vi "TrapControllers.vi"() -> ()   [LabVIEW 2016]
doc: "I. Description:\nThis example demonstrates how to continuously output a waveform using an internal sample clock. The automatic regeneration of data has been disabled, so new data has to be provided throughout the duration of the continuous Analog Output operation. This allows the generation of any arbitrary frequency as this VI computes new data for each iteration of the loop, maintaining phase continuity of the signal. The regeneration of data has also been adjusted so that the newest data is output as quickly as possible; thus reducing the lag between the changing of the data and the output of that data.\n\nII. Instructions for Running:\n1. Select the Physical Channel to correspond to where your signal is output on the DAQ device.\n2. Enter the Minimum and Maximum Voltage range.\n3. Specify the desired Sample Clock Rate of the output Waveform. Higher sample clock rates will produce a smoother waveform.\n4. Manually specify the Analog Output buffer size, in number of samples. A larger buffer would help non-regenerative operations avoid errors due to occasional high CPU load. \nNote: \nThe Analog Output buffer has to be at least as big as the amount of data being written to the board per iteration. The recommended buffer size would be at least twice the amount of data being written to the board per iteration.\n5. Enter the Waveform Information. See the documentation of the Basic Function Generator SubVI for information on each parameter.\n\nIII. Block Diagram Steps:\n1. Create an Analog Output Voltage channel.\n2. Configure the task to prohibit the automatic regeneration of data.\n2a. Set the transfer condition to Less than Full. Allows for more rapid updates of Output Buffer.\n3. Call the DAQmx (Sample Clock) VI to set the sample clock rate. Additionally, set the sample mode to Continuous.\n4. Read the actual sample clock rate (eventually coerced depending on the hardware used). \n5. Compute the desired waveform, using the buffer size and the actual update rate. This VI keeps track of the phase of the waveform to ensure that the generated signal is continuous.\n6. Write the waveform to the output buffer. \n7a. Call the Start VI. This is only needed when the loop is executed for the first time.\n7b. Do nothing.\n8. Loop continuously until user presses the Stop button. Every iteration computes and writes a new waveform to the buffer.\n9. Call the Clear Task VI to clear the Task.\n10. Use the popup dialog box to display an error or warning if any.\n\nIV. I/O Connections Overview:\nMake sure your signal output terminal matches the Physical Channel I/O Control. For further connection information, refer to your hardware reference manual."
uses:
  <vilib>/event_ctls.llb/eventvkey.ctl
  <vilib>/DAQmx/write.llb/DAQmx Write (Digital 1D Bool NChan 1Samp 1Line).vi
  <vilib>/DAQmx/write.llb/DAQmx Write (Analog DBL 1Chan 1Samp).vi
  <vilib>/DAQmx/write.llb/DAQmx Write (Analog 1D DBL NChan 1Samp).vi
  <vilib>/DAQmx/create/channels.llb/DAQmx Create Channel (DO-Digital Output).vi
  <vilib>/DAQmx/miscellaneous.llb/DAQmx Fill In Error Info.vi
  <vilib>/DAQmx/create/channels.llb/DAQmx Create Channel (AO-Voltage-Basic).vi
  PZT_PI/PZT_oscillation.vi
panel:
  in  "VISA resource name":refnum<visa-resource-name>
  out "Off":string
  out "Error 2":string
  out "On":string
  out "Move":string
  in  "Move":bool
  in  "Query?":bool
  in  "Step":i32 min=0 max=10 step=1
  out "Status":string
  out "Position":string
  out "Error":string
  in  "StageZ_Start":bool
  in  "StageY_Start":bool
  out "StageY_Connection":bool
  in  "StageY_Home":bool
  out "StageY_Position":dbl caption="Pos (um)" format="%.1f"
  in  "StageY_Step2":dbl=1.0 caption="Step2" min=0.0 max=1000.0 step=0.1 format="%.1f"
  in  "StageY_Step1":dbl=10.0 caption="Step1" min=0.0 max=1000.0 step=0.1 format="%.1f"
  out "StageY_Step":dbl=10.0 caption="Step (um)" min=0.0 max=1000.0 step=0.1 format="%.1f"
  out "VKey":T1
  out "Char":i16
  out "ScanCode":i16
  out "StageX_Step":dbl=10.0 caption="Step (um)" min=0.0 max=1000.0 step=0.1 format="%.1f"
  in  "StageX_Step2":dbl=1.0 caption="Step2" min=0.0 max=1000.0 step=0.1 format="%.1f"
  in  "Stage_Step_Select":bool=TRUE
  out "Numeric":i32
  out "StageX_Connection":bool
  in  "StageZ_Stop":bool
  in  "StageY_Stop":bool
  in  "StageX_Stop":bool
  in  "StageZ-":bool
  in  "StageZ+":bool
  in  "StageY-":bool
  in  "StageY+":bool
  in  "StageX+":bool
  in  "StageX-":bool
  out "StageY_Limit 2":bool caption="Limit"
  out "StageY_Limit":bool caption="Limit"
  out "StageX_Limit":bool caption="Limit"
  out "PZT_Error 6":bool
  out "PZT_Error 5":bool
  out "PZT_Error 4":bool
  out "PZT_Error 3":bool
  out "PZT_Error 2":bool
  out "PZT_Error":bool
  in  "StageX_Step1":dbl=10.0 caption="Step1" min=0.0 max=1000.0 step=0.1 format="%.1f"
  in  "StageX_Home":bool
  out "?":i32
  out "?":i32
  out "PZT_Z 2":dbl caption="Z"
  out "StageX_Position":dbl caption="Pos (um)" format="%.1f"
  in  "StageX_Start":bool
  in  "PZT_Step":dbl=10.0 caption="Step (nm)" min=0.0 max=1000.0 step=1.0
  in  "Flu_Red_Power":dbl=1.0 caption="(%)" min=0.0 max=100.0 step=1.0
  in  "Flu_Green_Power":dbl=1.0 caption="(%)" min=0.0 max=100.0 step=1.0
  in  "Flu_Blue_Power":dbl=1.0 caption="(%)" min=0.0 max=100.0 step=1.0
  in  "Flu_Red":bool caption="640"
  in  "Flu_Green":bool caption="561"
  in  "Flu_Blue":bool caption="488"
  in  "stop 6":bool
  out "Numeric 9":i32
  out "OK Button 10":bool
  in  "OK Button 6":bool
  in  "Trap_control 2":dbl=1.0 caption="Power (%)" min=1.0 max=10.0 step=0.1 format="%.1f"
  in  "Detection_Feedback":bool caption="Feedback"
  in  "Detection_ON":bool caption="ON/OFF (d)"
  in  "stop 4":bool
  out "Numeric 7":i32
  in  "OK Button 4":bool
  out "OK Button 8":bool
  in  "stop 5":bool
  out "Numeric 8":i32
  in  "OK Button 5":bool
  out "OK Button 9":bool
  in  "Trap_Feedback":bool caption="Feedback"
  in  "Trap_ON":bool caption="ON/OFF (t)"
  in  "Trap_control":dbl=1.0 caption="Power (%)" min=1.0 max=100.0 step=1.0
  in  "Trap_STOP1":bool
  out "Numeric 5":i32
  in  "Trap_START1":bool
  out "Trap_START2":bool
  in  "PZT_oscillation":bool caption="Start\n(Ctrl)"
  out "PZT_os_num":i32
  out "PZT_manual":bool
  in  "PZT_Amplitude":dbl=10.0 caption="Amp (nm)" min=0.0 max=100.0 step=1.0
  in  "PZT_Frequency":dbl=1.0 caption="Freq (Hz)" min=0.0 max=100.0 step=1.0
  in  "PZT_Waveform":T2(ring) caption="Waveform"
  in  "PZT_Axis":enum16{"X-axis", "Y-axis", "Z-axis"}(ring) caption="Axis"
  in  "PZTZ_move":dbl caption="Z" min=-3000.0 max=3000.0 step=1.0
  in  "PZTY_move":dbl caption="Y" min=-5000.0 max=5000.0 step=1.0
  in  "PZTX_move":dbl caption="X" min=-5000.0 max=5000.0 step=1.0
  out "PZTZ_Vin":dbl format="%.5f"
  out "PZTY_Vin":dbl format="%.5f"
  out "PZTX_Vin":dbl format="%.5f"
  out "PZT_Z":dbl caption="Z"
  out "PZT_Y":dbl caption="Y"
  out "PZT_X":dbl caption="X"
  in  "PZT_Move":bool
  out "PZT_Caution":bool caption="Limit"
  in  "PZT_Time":dbl=100.0 caption="Vel (%)" min=0.0 max=100.0 step=1.0
  in  "PZT_Center":bool
  in  "PZT_Z-":bool
  in  "PZT_Z+":bool
  in  "PZT_Y-":bool
  in  "PZT_Y+":bool
  in  "PZT_X+":bool
  in  "PZT_X-":bool
  out "PZT_ON":bool
  in  "PZT_START":bool
  out "PZT_man_num":i32
  in  "PZT_STOP":bool
  in  "STOP":bool
  # "Stop sub-programs first >> STOP PROGRAM"
  # "Servo should be ON.\nProgram START -> PZT power ON\nRange: X/Y = +/- 5 um, Z = +/- 3 um"
  # "Stage"
  # "PZT"
  # "Range: X/Y = +/- 2.5 mm"
  # "Move to"
  # "Pos (nm)"
  # "Vin (V)"
  # "Manual"
  # "Oscillation"
  # "Feedback"
  # "1 = 10 nm"
  # "Trap Laser"
  # "Detection Laser"
  # "Fluorescent Laser"
  # "Template"
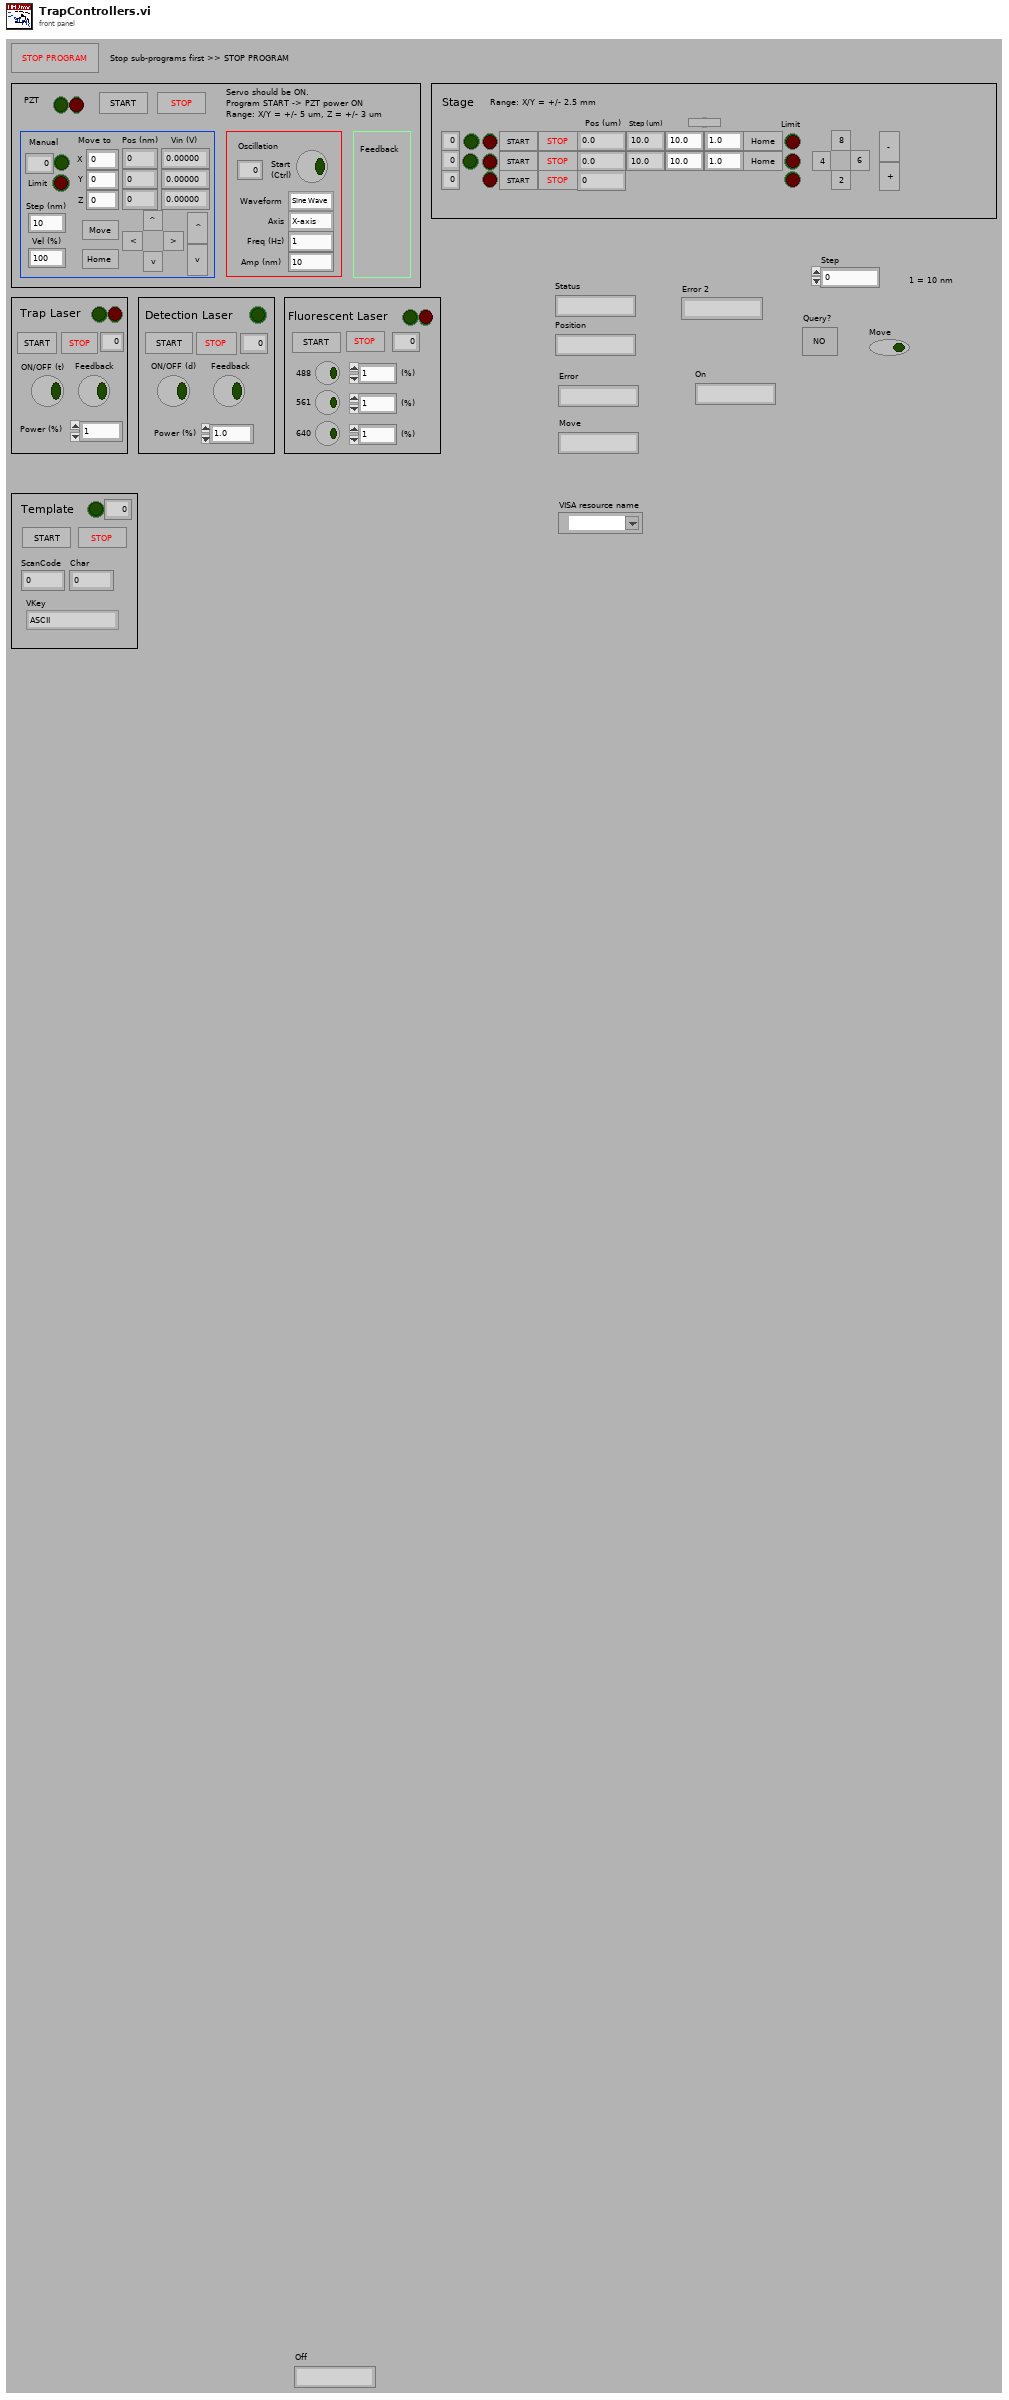
[diagram p1: front panel]
types:
  T1 = typedef "eventvkey.ctl" = enum16{"ASCII", "Enter", "Return", "Shift", "Ctrl", "Alt", "Cmd", "Opt", "Caps", "NumLock", "Clear", "Break", "Up", "Down", "Left", "Right", "Insert", "Delete", "Home", "End", "PageUp", "PageDown", "Escape", "Help", "Pause", "ScrollLock", "F1", "F2", "F3", "F4", "F5", "F6", "F7", "F8", "F9", "F10", "F11", "F12", "F13", "F14", "F15", "F16", "F17", "F18", "F19", "F20", "F21", "F22", "F23", "F24", "Play", "VolumeUp", "VolumeDown", "Mute", "Two Byte Char"}
  T2 = enum16{"Sine Wave", "Triangle Wave", "Square Wave", "Sawtooth Wave"}
  T3 = cluster{"VISA resource name":refnum<visa-resource-name>, "Device name":string, "Controller address":i32, "error":errorcluster}
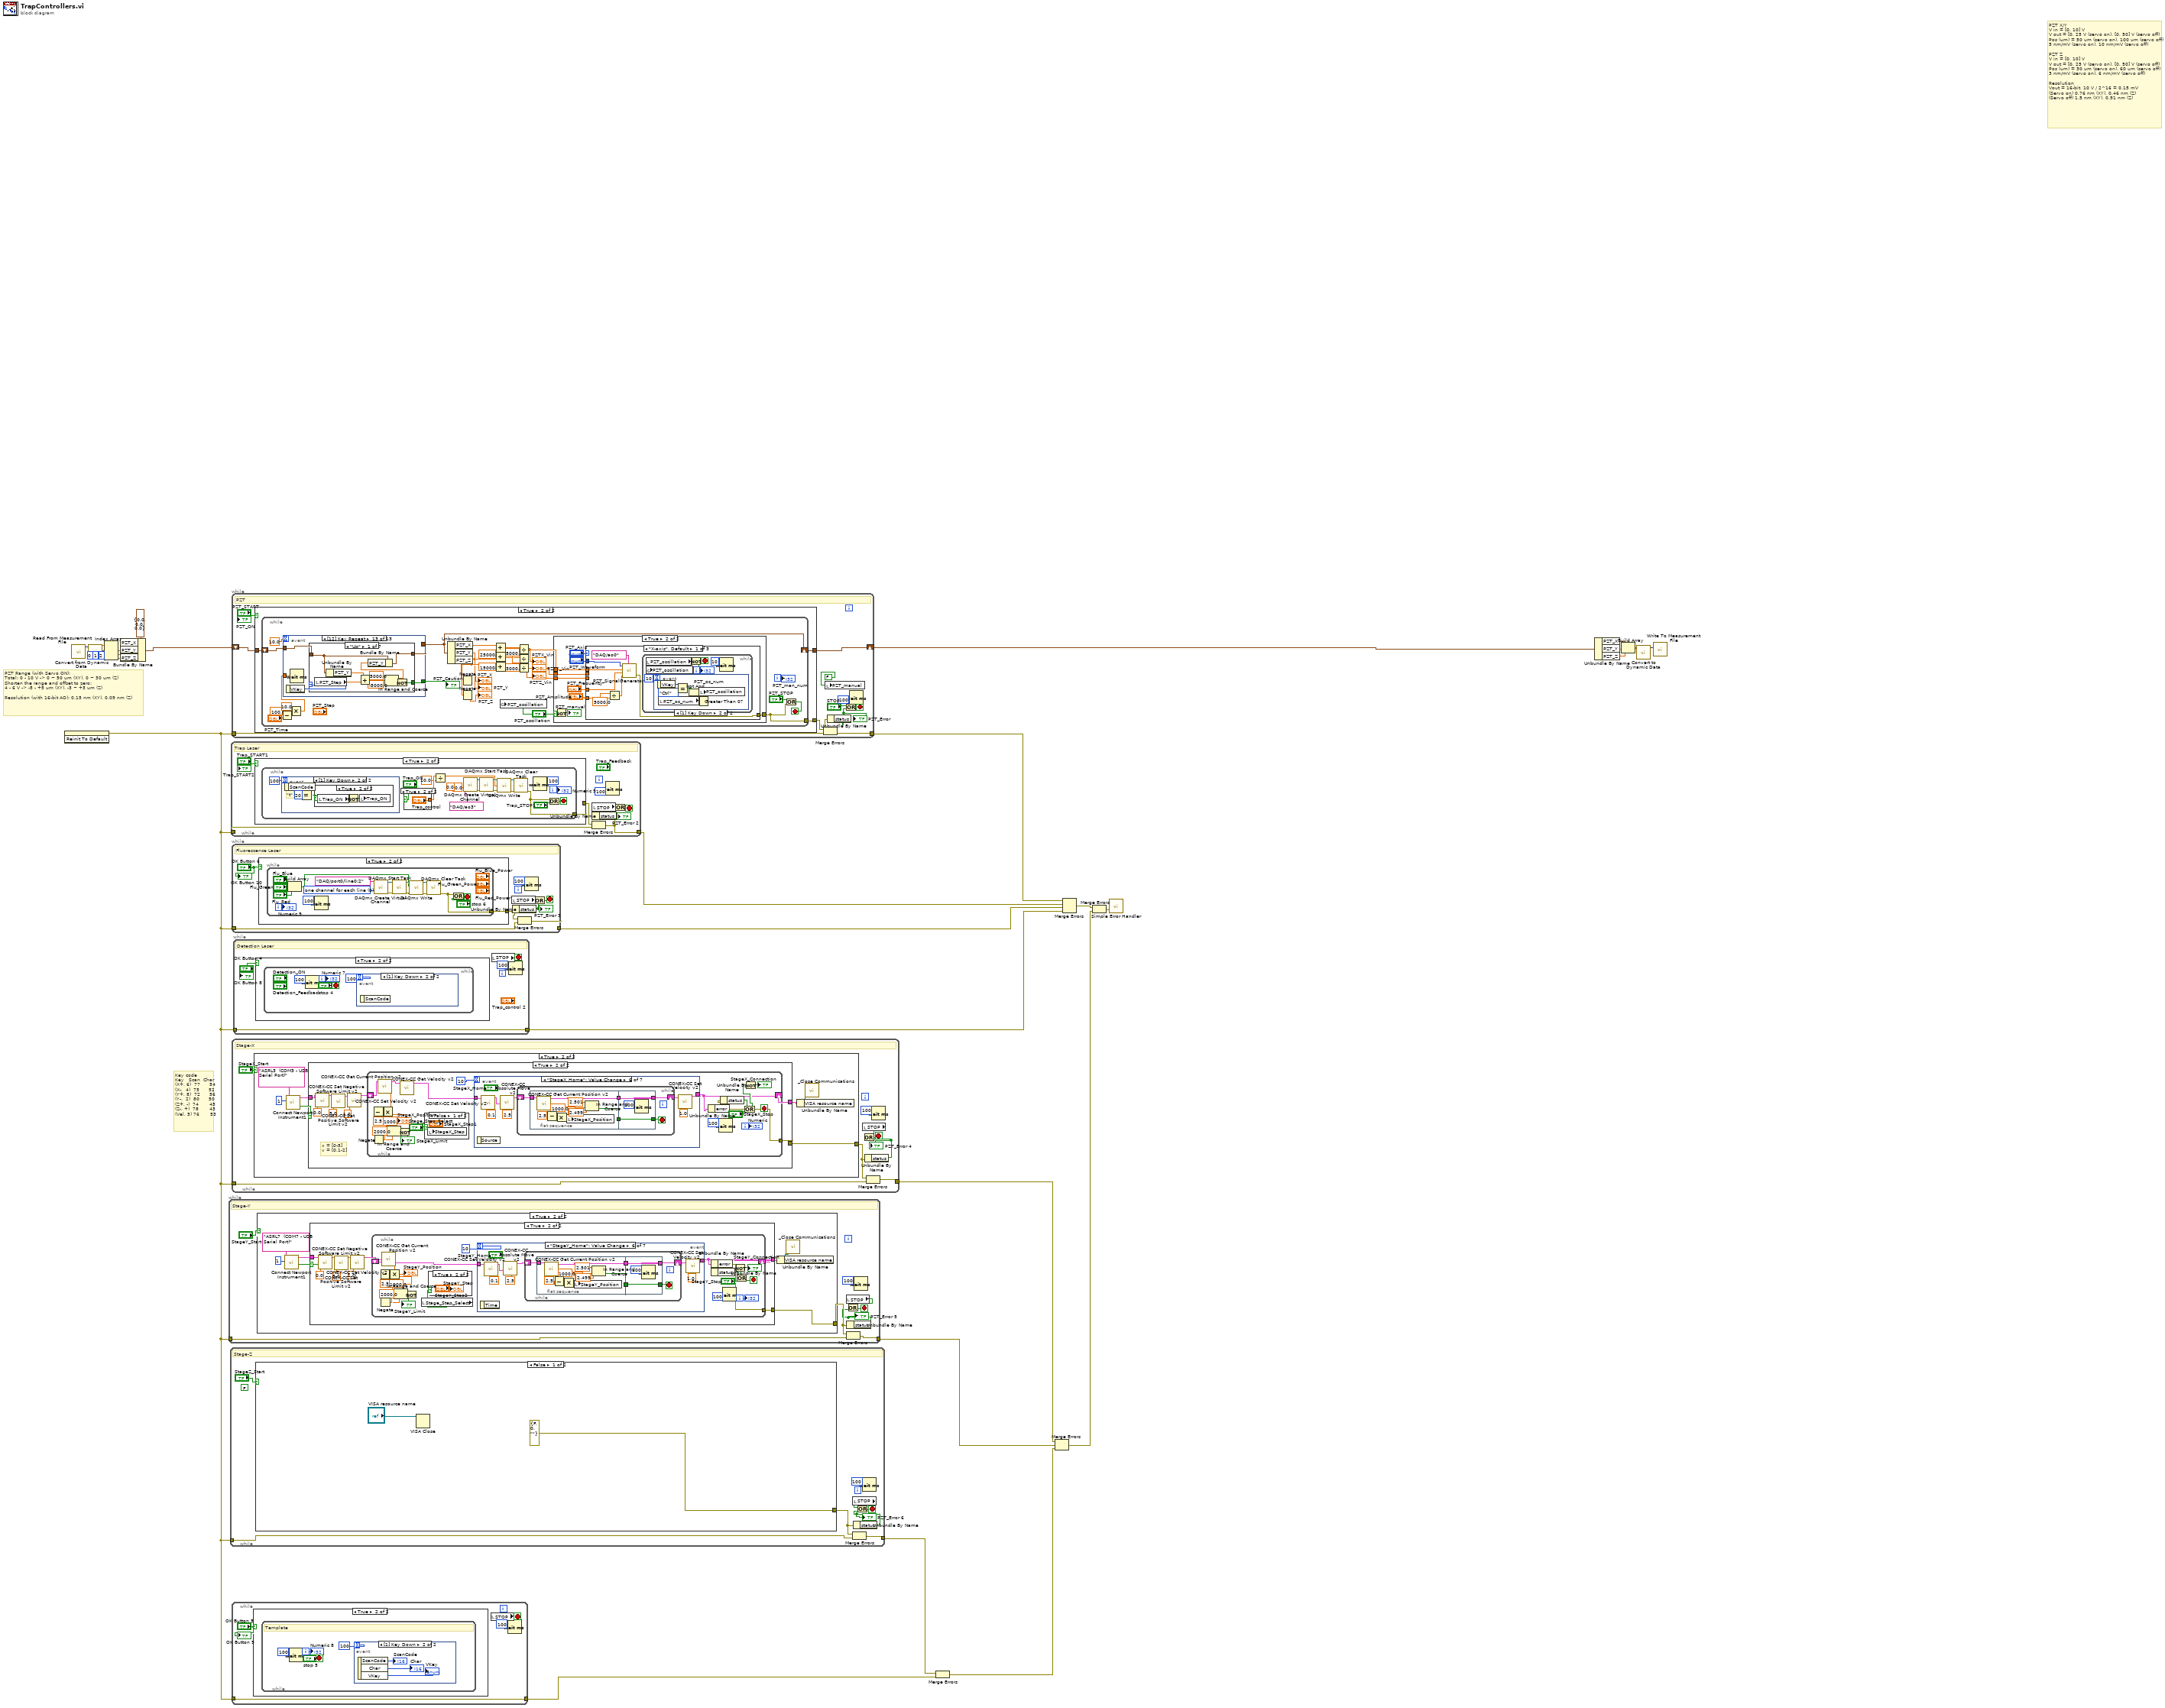
[diagram p0: block diagram]
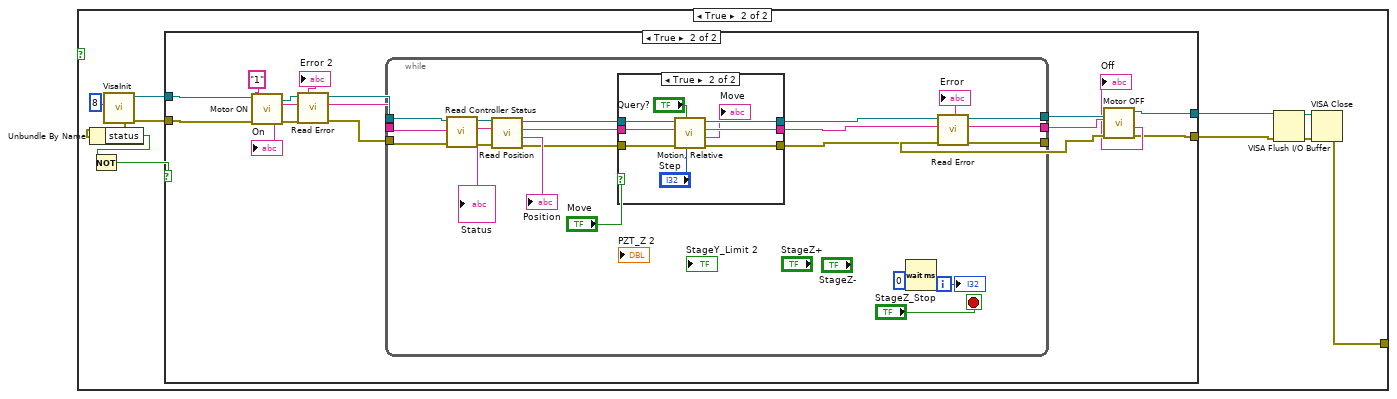
[diagram p2: hidden frame]
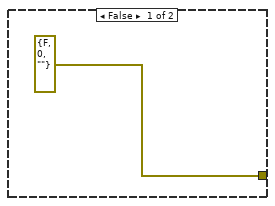
[diagram p5: hidden frame]
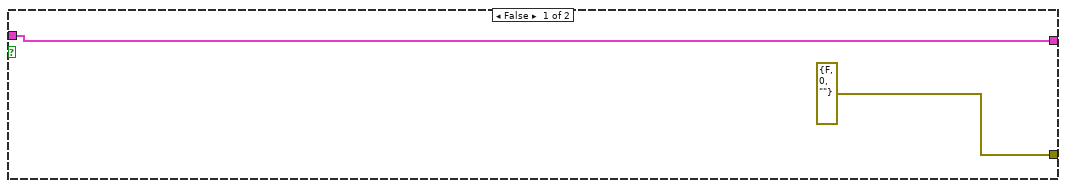
[diagram p6: hidden frame]
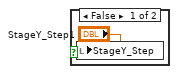
[diagram p7: hidden frame]
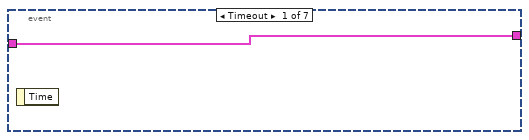
[diagram p8: hidden frame]
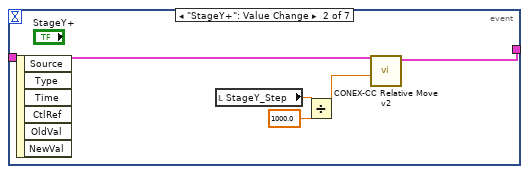
[diagram p9: hidden frame]
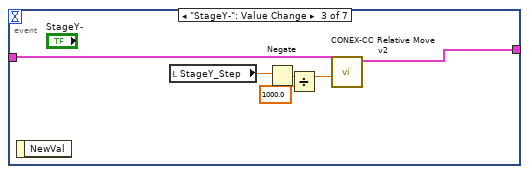
[diagram p10: hidden frame]
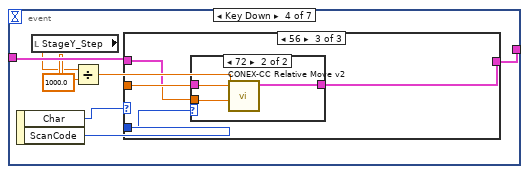
[diagram p11: hidden frame]
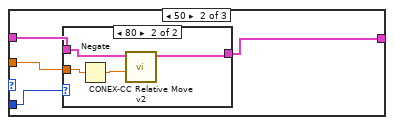
[diagram p13: hidden frame]
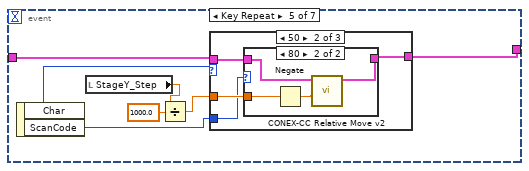
[diagram p16: hidden frame]
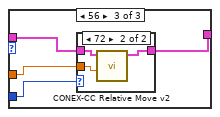
[diagram p19: hidden frame]
diagram:
  # "Key code\nKey   Scan  Char\n(X+, 6)  77      54\n(X-,  4)  75      52\n(Y+, 8)  72      56\n(Y-,  2)  80      50\n(Z+, -)  74       45\n(Z-, +)  78       43\n(Vel, 5) 76       53"
  # "PZT Range (with Servo ON):\nTotal: 0 - 10 V -> 0 ~ 50 um (XY), 0 ~ 30 um (Z)\nShorten the range and offset to zero: \n4 - 6 V -> -5 - +5 um (XY), -3 ~ +3 um (Z)\n\nResolution (with 16-bit AO): 0.15 nm (XY), 0.09 nm (Z)"
  # "PZT X/Y\nV in = [0, 10] V\nV out = [0, 25 V (servo on), [0, 50] V (servo off)\nPos (um) = 50 um (servo on), 100 um (servo off)\n5 nm/mV (servo on), 10 nm/mV (servo off)\n\nPZT Z\nV in = [0, 10] V\nV out = [0, 25 V (servo on), [0, 50] V (servo off)\nPos (um) = 30 um (servo on), 60 um (servo off)\n3 nm/mV (servo on), 6 nm/mV (servo off)\n\nResolution\nVout = 16-bit, 10 V / 2^16 = 0.15 mV\n(Servo on) 0.76 nm (XY), 0.46 nm (Z)\n(Servo off) 1.5 nm (XY), 0.91 nm (Z)"
  n1 = invoke on="STOP" class="Bool (strict)" method="Reinit To Default"() -> (error out=w2:errorcluster)  [unwired: 3 in, 2 out]
  n2 = call "Read From Measurement File"() -> ("Signals"=w26:dynamicdata)  [unwired: 6 in, 5 out]
  n3 = call "Convert from Dynamic Data"("Dynamic Data Type"=w26) -> ("Array"=w25:dbl[])  [unwired: 3 in]
  n4 = Index Array(array=w25, index #1=0 ("index"), index #2=1 ("index"), index #3=2 ("index")) -> (element #1=w21:dbl, element #2=w20:dbl, element #3=w19:dbl)
  n5 = Bundle By Name(cluster=cluster{"PZT_X":dbl, "PZT_Y":dbl, "PZT_Z":dbl} {"PZT_X"=0.0, "PZT_Y"=0.0, "PZT_Z"=0.0} ("output cluster"), "PZT_X"=w21, "PZT_Y"=w20, "PZT_Z"=w19) -> (w12:cluster{"PZT_X":dbl, "PZT_Y":dbl, "PZT_Z":dbl})
  n6 = while {
    tunnel: w2 -> [w36]
    tunnel: [w35] -> w9
    stop <- w32 stop-if-true
    # "Stage-Y"
    n7 = case shown="True" "StageY_Start" {
      tunnel: [errorcluster {"status"=FALSE, "code"=0, "source"=""} ("error out") w40] -> w34
      frame False {
      }
      frame True {
        n8 = call <userlib>:"Connect Newport Instrument1.vi"("Controller address"=1, "Selected device"="ASRL7  (COM7 - USB Serial Port)" ("String")) -> ("Connected"=w44:bool, "Device Connection Cluster"=w43:T3)  [unwired: 5 in, 3 out]
        n9 = case shown="True" w44 {
          tunnel: w43 -> [w47 w51]
          tunnel: [w47 w50] -> w41
          tunnel: [errorcluster {"status"=FALSE, "code"=0, "source"=""} ("error") w49] -> w40
          frame False {
          }
          frame True {
            n10 = call <userlib>:"CONEX-CC Set Negative Software Limit v2.vi"("Negative limit (left)"=0.0, "Connection Cluster in"=w51) -> ("Connection Cluster out"=w56:T3)  [unwired: 9 in]
            n11 = call <userlib>:"CONEX-CC Set Positive Software Limit v2.vi"("Positive limit (right)"=5.0, "Connection Cluster in"=w56) -> ("Connection Cluster out"=w55:T3)  [unwired: 9 in]
            n12 = call <userlib>:"CONEX-CC Set Velocity v2.vi"("Velocity"=1.0, "Connection Cluster in"=w55) -> ("Connection Cluster out"=w48:T3)  [unwired: 9 in]
            n13 = while "Event Handle Loop" {
              shift-right: [w64] -> w50
              shift-left: w48 -> [w68]
              tunnel: [w59] -> w49
              i -> [w76]
              stop <- w61 stop-if-true
              w74 = 2000.0 ("upper limit")
              # "Stage-Y"
              n14 = Negate(x=w74) -> (-x=w75:dbl)
              n15 = call <userlib>:"CONEX-CC Get Current Position v2.vi"("Connection Cluster in"=w68) -> ("Current position"=w69:dbl, "Connection Cluster out"=w66:T3)  [unwired: 8 in, 1 out]
              n16 = Subtract(x=w69, y=2.5) -> (x-y=w71:dbl)
              n17 = Multiply(x=w71, y=1000.0) -> (x*y=w58:dbl)
              "StageY_Position" <- w58
              n18 = In Range and Coerce(upper limit=w74, x=w58, lower limit=w75) -> (In Range?=w73:bool)  [unwired: 1 out]
              n19 = Not(x=w73) -> (.not. x?=→"StageY_Limit":bool)
              n20 = local read "Stage_Step_Select"() -> (w57:bool)
              n21 = case shown="True" w57 {
                frame False {
                  n22 = local write "StageY_Step"("StageY_Step1") -> ()
                }
                frame True {
                  "StageY_Step" <- "StageY_Step2"
                }
              }
              n23 = event shown="[5] \"StageY_Home\": Value Change" {
                selector: _ -> [_ _ _ _ _ _ _]
                dyn-events: _ -> [_ _ _ _ _ _ _]
                timeout: 10 -> [_ _ _ _ _ _ _]
                tunnel: w66 -> [w80 w81 w91 w98 w123 w149 w171]
                tunnel: [w80 w85 w88 w97 w122 w142 w171] -> w64
                event Timeout {
                  n24 = event-data() -> ()  [unwired: 1 in, 1 out]
                }
                event "StageY+": Value Change {
                  n25 = event-data() -> ()  [unwired: 1 in, 6 out]
                  n26 = local read "StageY_Step"() -> (w82:dbl)
                  n27 = Divide(x=w82, y=1000.0) -> (x/y=w84:dbl)
                  n28 = call <userlib>:"CONEX-CC Relative Move v2.vi"("Relative displacement"=w84, "Connection Cluster in"=w81) -> ("Connection Cluster out"=w85:T3)  [unwired: 9 in]
                }
                event "StageY-": Value Change {
                  n29 = event-data() -> ()  [unwired: 1 in, 1 out]
                  n30 = local read "StageY_Step"() -> (w90:dbl)
                  n31 = Negate(x=w90) -> (-x=w89:dbl)
                  n32 = Divide(x=w89, y=1000.0) -> (x/y=w87:dbl)
                  n33 = call <userlib>:"CONEX-CC Relative Move v2.vi"("Relative displacement"=w87, "Connection Cluster in"=w91) -> ("Connection Cluster out"=w88:T3)  [unwired: 9 in]
                }
                event Key Down {
                  n34 = event-data() -> ("Char"=w93:i16, "ScanCode"=w92:i16)  [unwired: 1 in]
                  n35 = local read "StageY_Step"() -> (w95:dbl)
                  n36 = Divide(x=w95, y=1000.0) -> (x/y=w94:dbl)
                  n37 = case shown="56" w93 {
                    tunnel: w98 -> [w99 w103 w112]
                    tunnel: [w99 w102 w111] -> w97
                    tunnel: w94 -> [_ w101 w110]
                    tunnel: w92 -> [_ w100 w109]
                    frame 0, Default {
                    }
                    frame 50 {
                      n38 = case shown="80" w100 {
                        tunnel: w103 -> [w104 w108]
                        tunnel: [w104 w107] -> w102
                        tunnel: w101 -> [_ w106]
                        frame 0, Default {
                        }
                        frame 80 {
                          n39 = Negate(x=w106) -> (-x=w105:dbl)
                          n40 = call <userlib>:"CONEX-CC Relative Move v2.vi"("Relative displacement"=w105, "Connection Cluster in"=w108) -> ("Connection Cluster out"=w107:T3)  [unwired: 9 in]
                        }
                      }
                    }
                    frame 56 {
                      n41 = case shown="72" w109 {
                        tunnel: w112 -> [w113 w116]
                        tunnel: [w113 w115] -> w111
                        tunnel: w110 -> [_ w114]
                        frame 0, Default {
                        }
                        frame 72 {
                          n42 = call <userlib>:"CONEX-CC Relative Move v2.vi"("Relative displacement"=w114, "Connection Cluster in"=w116) -> ("Connection Cluster out"=w115:T3)  [unwired: 9 in]
                        }
                      }
                    }
                  }
                }
                event Key Repeat {
                  n43 = event-data() -> ("Char"=w121:i16, "ScanCode"=w117:i16)  [unwired: 1 in]
                  n44 = local read "StageY_Step"() -> (w119:dbl)
                  n45 = Divide(x=w119, y=1000.0) -> (x/y=w118:dbl)
                  n46 = case shown="50" w121 {
                    tunnel: w123 -> [w124 w128 w137]
                    tunnel: [w124 w127 w136] -> w122
                    tunnel: w118 -> [_ w126 w135]
                    tunnel: w117 -> [_ w125 w134]
                    frame 0, Default {
                    }
                    frame 50 {
                      n47 = case shown="80" w125 {
                        tunnel: w128 -> [w129 w133]
                        tunnel: [w129 w132] -> w127
                        tunnel: w126 -> [_ w131]
                        frame 0, Default {
                        }
                        frame 80 {
                          n48 = Negate(x=w131) -> (-x=w130:dbl)
                          n49 = call <userlib>:"CONEX-CC Relative Move v2.vi"("Relative displacement"=w130, "Connection Cluster in"=w133) -> ("Connection Cluster out"=w132:T3)  [unwired: 9 in]
                        }
                      }
                    }
                    frame 56 {
                      n50 = case shown="72" w134 {
                        tunnel: w137 -> [w138 w141]
                        tunnel: [w138 w140] -> w136
                        tunnel: w135 -> [_ w139]
                        frame 0, Default {
                        }
                        frame 72 {
                          n51 = call <userlib>:"CONEX-CC Relative Move v2.vi"("Relative displacement"=w139, "Connection Cluster in"=w141) -> ("Connection Cluster out"=w140:T3)  [unwired: 9 in]
                        }
                      }
                    }
                  }
                }
                event "StageY_Home": Value Change {
                  n52 = event-data() -> ()  [unwired: 1 in, 1 out]
                  n53 = call <userlib>:"CONEX-CC Set Velocity v2.vi"("Velocity"=0.1, "Connection Cluster in"=w149) -> ("Connection Cluster out"=w148:T3)  [unwired: 9 in]
                  n54 = call <userlib>:"CONEX-CC Absolute Move v2.vi"("Target position"=2.5, "Connection Cluster in"=w148) -> ("Connection Cluster out"=w145:T3)  [unwired: 5 in, 2 out]
                  n55 = while {
                    shift-right: [w150] -> w143
                    shift-left: w145 -> [w154]
                    stop <- w152 stop-if-true
                    n56 = flat-sequence {
                      tunnel: w154 -> [w162]
                      tunnel: [w161] -> w153
                      tunnel: [w160] -> w151
                      tunnel: w153 -> [w166]
                      tunnel: [w166] -> w152
                      tunnel: w151 -> [w165]
                      tunnel: [w165] -> w150
                      frame #0 {
                        n57 = call <userlib>:"CONEX-CC Get Current Position v2.vi"("Connection Cluster in"=w162) -> ("Current position"=w159:dbl, "Connection Cluster out"=w160:T3)  [unwired: 8 in, 1 out]
                        n58 = Subtract(x=w159, y=2.5) -> (x-y=w158:dbl)
                        n59 = Multiply(x=1000.0, y=w158) -> (x*y=w156:dbl)
                        n60 = local write "StageY_Position"(w156) -> ()
                        n61 = In Range and Coerce(upper limit=2.501 ("x"), x=w159, lower limit=2.499 ("x")) -> (In Range?=w161:bool)  [unwired: 1 out]
                      }
                      frame #1 {
                        n62 = Wait (ms)(milliseconds to wait=u32 100) -> ()  [unwired: 1 out]
                      }
                    }
                  }
                  n63 = call <userlib>:"CONEX-CC Set Velocity v2.vi"("Velocity"=1.0, "Connection Cluster in"=w143) -> ("Connection Cluster out"=w142:T3)  [unwired: 9 in]
                }
                event "Stage_Step_Select": Value Change {
                  n64 = event-data() -> ()  [unwired: 1 in, 1 out]
                  n65 = local read "Stage_Step_Select"() -> (w169:bool)
                  n66 = local read "StageY_Step1"() -> (w168:dbl)
                  n67 = local read "StageY_Step2"() -> (w170:dbl)
                  n68 = Select(t=w170, s=w169, f=w168) -> (s? t:f=w172:dbl)
                  n69 = local write "StageY_Step"(w172) -> ()
                }
              }
              n70 = Unbundle By Name(w64) -> ("error"=w59:errorcluster)
              n71 = Unbundle By Name(w59) -> ("status"=w62:bool)
              n72 = Wait (ms)(milliseconds to wait=u32 100) -> ()  [unwired: 1 out]
              n73 = Or(x=w62, y="StageY_Stop") -> (x .or. y?=w61:bool)
              n74 = Not(x=w61) -> (.not. x?=→"StageY_Connection":bool)
              "?" <- w76
            }
          }
        }
        n75 = Unbundle By Name(w41) -> ("VISA resource name"=w42:refnum<visa-resource-name>)
        n76 = call <userlib>:"_Close Communications.vi"("Instrument Channel"=w42) -> ()  [unwired: 14 in, 1 out]
      }
    }
    n77 = local read "STOP"() -> (w33:bool)
    n78 = Merge Errors(w34, w36) -> (w35:errorcluster)
    n79 = Unbundle By Name(w34) -> ("status"=w31:bool)
    "PZT_Error 5" <- w31
    n80 = Or(x=w33, y=w31) -> (x .or. y?=w32:bool)
    n81 = Wait (ms)(milliseconds to wait=u32 100) -> ()  [unwired: 1 out]
  }
  n82 = while {
    tunnel: w2 -> [w179]
    tunnel: [w178] -> w4
    stop <- w176 stop-if-true
    (unwired) FALSE
    # "Stage-Z"
    n83 = case shown="False" "StageZ_Start" {
      tunnel: [errorcluster {"status"=FALSE, "code"=0, "source"=""} ("error out") w187] -> w177
      frame False {
        n84 = VISA Close(VISA resource name="VISA resource name") -> ()  [unwired: 1 in, 1 out]
      }
      frame True {
        n85 = call <userlib>:"VisaInit.vi"("SerialPort"=u8 8) -> ("error out"=w185:errorcluster, "Visa Handle"=w186:refnum<visa-resource-name>)  [unwired: 6 in]
        n86 = Unbundle By Name(w185) -> ("status"=w191:bool)
        n87 = Not(x=w191) -> (.not. x?=w190:bool)
        n88 = case shown="True" w190 {
          tunnel: [w193 w195] -> w184
          tunnel: [w194 w196] -> w183
          tunnel: w186 -> [w194 w202]
          tunnel: w185 -> [w193 w201]
          frame False {
          }
          frame True {
            n89 = call <userlib>:"Motor ON.vi"("error in (no error)"=w201, "Controller #"="1", "VISA Handle"=w202) -> ("error out"=w208:errorcluster, "Response"=→"On":string, "Dup Controller #"=w209:string, "Dup VISA Handle"=w207:refnum<visa-resource-name>)  [unwired: 2 in, 1 out]
            n90 = call <userlib>:"Read Error.vi"("error in (no error)"=w208, "Controller #"=w209, "VISA Handle"=w207) -> ("error out"=w203:errorcluster, "Response"=→"Error 2":string, "Dup Controller #"=w204:string, "Dup VISA Handle"=w205:refnum<visa-resource-name>)  [unwired: 2 in, 1 out]
            n91 = while "Event Handle Loop" {
              tunnel: w205 -> [w230]
              tunnel: w203 -> [w228]
              tunnel: [w214] -> w198
              tunnel: w204 -> [w229]
              tunnel: [w213] -> w199
              tunnel: [w212] -> w200
              i -> [w232]
              stop <- "StageZ_Stop" stop-if-true
              # "Stage-Z"
              n92 = call <userlib>:"Read Controller Status.vi"("error in (no error)"=w228, "Controller #"=w229, "VISA Handle"=w230) -> ("error out"=w225:errorcluster, "Response"=→"Status":string, "Dup Controller #"=w226:string, "Dup VISA Handle"=w227:refnum<visa-resource-name>)  [unwired: 2 in, 1 out]
              n93 = call <userlib>:"Read Position.vi"("error in (no error)"=w225, "Controller #"=w226, "VISA Handle"=w227) -> ("error out"=w220:errorcluster, "Response"=→"Position":string, "Dup Controller #"=w221:string, "Dup VISA Handle"=w222:refnum<visa-resource-name>)  [unwired: 2 in, 1 out]
              n94 = case shown="True" "Move" {
                tunnel: w222 -> [w236 w245]
                tunnel: [w236 w244] -> w217
                tunnel: w221 -> [w235 w243]
                tunnel: [w235 w242] -> w216
                tunnel: w220 -> [w234 w241]
                tunnel: [w234 w240] -> w215
                frame False {
                }
                frame True {
                  n95 = call <userlib>:"Motion, Relative.vi"("Value"="Step", "Query?"="Query?", "error in (no error)"=w241, "Controller #"=w243, "VISA Handle"=w245) -> ("error out"=w240:errorcluster, "Response"=→"Move":string, "Dup Controller #"=w242:string, "Dup VISA Handle"=w244:refnum<visa-resource-name>)  [unwired: 1 in, 1 out]
                }
              }
              n96 = Wait (ms)(milliseconds to wait=u32 0) -> ()  [unwired: 1 out]
              n97 = call <userlib>:"Read Error.vi"("error in (no error)"=w215, "Controller #"=w216, "VISA Handle"=w217) -> ("error out"=w212:errorcluster, "Response"=→"Error":string, "Dup Controller #"=w213:string, "Dup VISA Handle"=w214:refnum<visa-resource-name>)  [unwired: 2 in, 1 out]
              "?" <- w232
            }
            n98 = call <userlib>:"Motor OFF.vi"("error in (no error)"=w200, "Controller #"=w199, "VISA Handle"=w198) -> ("error out"=w195:errorcluster, "Response"=→"Off":string, "Dup VISA Handle"=w196:refnum<visa-resource-name>)  [unwired: 2 in, 2 out]
          }
        }
        n99 = VISA Flush I/O Buffer(VISA resource name=w183, error in (no error)=w184) -> (VISA resource name out=w189:refnum<visa-resource-name>, error out=w188:errorcluster)  [unwired: 1 in]
        n100 = VISA Close(VISA resource name=w189, error in (no error)=w188) -> (error out=w187:errorcluster)
      }
    }
    n101 = local read "STOP"() -> (w175:bool)
    n102 = Merge Errors(w177, w179) -> (w178:errorcluster)
    n103 = Unbundle By Name(w177) -> ("status"=w174:bool)
    "PZT_Error 6" <- w174
    n104 = Or(x=w175, y=w174) -> (x .or. y?=w176:bool)
    n105 = Wait (ms)(milliseconds to wait=u32 100) -> ()  [unwired: 1 out]
  }
  n106 = while {
    tunnel: w2 -> [w246]
    tunnel: [w248] -> w28
    stop <- w251 stop-if-true
    # "Trap Laser"
    n107 = case shown="True" "Trap_START1" {
      tunnel: [errorcluster {"status"=FALSE, "code"=0, "source"=""} ("error out") w255] -> w250
      frame False {
      }
      frame True {
        n108 = while "Event Handle Loop" {
          tunnel: [w269] -> w255
          i -> [w273]
          stop <- w271 stop-if-true
          # "Trap Laser"
          n109 = event shown="[1] Key Down" {
            selector: _ -> [_ _]
            dyn-events: _ -> [_ _]
            timeout: 100 -> [_ _]
            event Timeout {
              n110 = event-data() -> ()  [unwired: 1 in, 1 out]
            }
            event Key Down {
              # "\"t\""
              n111 = event-data() -> ("ScanCode"=w279:i16)  [unwired: 1 in]
              n112 = Equal?(x=i16 20, y=w279) -> (x = y?=w277:bool)
              n113 = case shown="True" w277 {
                frame False {
                }
                frame True {
                  n114 = local read "Trap_ON"() -> (w281:bool)
                  n115 = Not(x=w281) -> (.not. x?=w280:bool)
                  n116 = local write "Trap_ON"(w280) -> ()
                }
              }
            }
          }
          n117 = case shown="True" "Trap_ON" {
            tunnel: [0.0 ("Trap_control") "Trap_control"] -> w258
            frame False {
            }
            frame True {
            }
          }
          n118 = Divide(x=w258, y=10.0) -> (x/y=w257:dbl)
          n119 = call-poly <vilib>:"DAQmx Create Virtual Channel.vi"("maximum value"=10.0, "minimum value"=0.0, "physical channels"=tag "DAQ/ao3") -> ("task out"=w265:refnum<k21>, "error out"=w264:errorcluster)  [unwired: 11 in]
          n120 = call <vilib>:"DAQmx Start Task.vi"("task/channels in"=w265, "error in"=w264) -> ("task out"=w263:refnum<k21>, "error out"=w262:errorcluster)  [unwired: 12 in]
          n121 = call-poly <vilib>:"DAQmx Write.vi"("task/channels in"=w263, "data"=w257, "error in"=w262) -> ("task out"=w261:refnum<k21>, "error out"=w260:errorcluster)  [unwired: 10 in, 1 out]
          n122 = call <vilib>:"DAQmx Clear Task.vi"("task in"=w261, "error in"=w260) -> ("error out"=w269:errorcluster)  [unwired: 13 in]
          n123 = Wait (ms)(milliseconds to wait=u32 100) -> ()  [unwired: 1 out]
          n124 = Or(x=w269, y="Trap_STOP1") -> (x .or. y?=w271:bool)
          "Numeric 5" <- w273
        }
      }
    }
    n125 = Merge Errors(w250, w246) -> (w248:errorcluster)
    n126 = local read "STOP"() -> (w249:bool)
    n127 = Unbundle By Name(w248) -> ("status"=w247:bool)
    "PZT_Error 2" <- w247
    n128 = Wait (ms)(milliseconds to wait=u32 100) -> ()  [unwired: 1 out]
    n129 = Or(x=w249, y=w247) -> (x .or. y?=w251:bool)
    "Trap_START2" <- "Trap_START1"
  }
  n130 = while {
    tunnel: w2 -> [w282]
    tunnel: [w282] -> w1
    stop <- w285 stop-if-true
    n131 = case shown="True" "OK Button 5" {
      frame False {
      }
      frame True {
        n132 = while "Event Handle Loop" {
          i -> [w286]
          stop <- "stop 5" stop-if-true
          # "Template"
          n133 = Wait (ms)(milliseconds to wait=u32 100) -> ()  [unwired: 1 out]
          n134 = event shown="[1] Key Down" {
            selector: _ -> [_ _]
            dyn-events: _ -> [_ _]
            timeout: 100 -> [_ _]
            event Timeout {
              n135 = event-data() -> ()  [unwired: 1 in, 2 out]
            }
            event Key Down {
              n136 = event-data() -> ("ScanCode"=→"ScanCode":i16, "Char"=→"Char":i16, "VKey"=→"VKey":T1)  [unwired: 1 in]
            }
          }
          "Numeric 8" <- w286
        }
      }
    }
    n137 = local read "STOP"() -> (w285:bool)
    n138 = Wait (ms)(milliseconds to wait=u32 100) -> ()  [unwired: 1 out]
    "OK Button 9" <- "OK Button 5"
  }
  n139 = while "PZT_Loop" {
    shift-right: [w302] -> w15
    shift-left: w12 -> [w303]
    tunnel: [w294] -> w29
    tunnel: w2 -> [w298]
    stop <- w300 stop-if-true
    # "PZT"
    n140 = case shown="True" "PZT_START" {
      tunnel: w303 -> [w305 w308]
      tunnel: [w305 w307] -> w302
      tunnel: [errorcluster {"status"=FALSE, "code"=0, "source"=""} ("error out") w306] -> w299
      frame False {
      }
      frame True {
        n141 = while "Event Handle Loop" {
          shift-right: [w331] -> w307
          shift-left: w308 -> [w332]
          tunnel: [w317] -> w306
          i -> [w337]
          stop <- w327 stop-if-true
          w322 = 25000.0 ("y")
          w334 = 5000.0 ("y")
          # "PZT"
          n142 = Subtract(x=100.0, y="PZT_Time") -> (x-y=w313:dbl)
          n143 = Multiply(x=10.0, y=w313) -> (x*y=w310:dbl)
          n144 = event shown="[12] Key Repeat" {
            selector: _ -> [_ _ _ _ _ _ _ _ _ _ _ _ _]
            dyn-events: _ -> [_ _ _ _ _ _ _ _ _ _ _ _ _]
            timeout: 10.0 -> [_ _ _ _ _ _ _ _ _ _ _ _ _]
            tunnel: w332 -> [w422 w431 w442 w453 w464 w475 w486 w492 w498 w502 w569 w575 w584]
            tunnel: [w422 w432 w443 w454 w465 w476 w487 w491 w497 w501 _ _ w583] -> w331
            tunnel: [FALSE w425 w438 w448 w461 w469 w480 _ _ w500 _ _ w582] -> w335
            tunnel: w310 -> [_ w424 w435 w446 w457 w468 w479 w490 w493 w499 _ _ w581]
            event Timeout {
              n145 = event-data() -> ()  [unwired: 1 in, 1 out]
            }
            event "PZT_X+": Value Change {
              n146 = event-data() -> ()  [unwired: 1 in, 1 out]
              n147 = Wait (ms)(milliseconds to wait=w424) -> ()  [unwired: 1 out]
              n148 = local read "PZT_Step"() -> (w423:dbl)
              n149 = Unbundle By Name(w431) -> ("PZT_X"=w433:dbl)
              n150 = Subtract(x=w433, y=w423) -> (x-y=w428:dbl)
              n151 = In Range and Coerce(upper limit=5000.0, x=w428, lower limit=-5000.0) -> (coerced(x)=w427:dbl, In Range?=w426:bool)
              n152 = Bundle By Name(cluster=w431, "PZT_X"=w427) -> (w432:cluster{"PZT_X":dbl, "PZT_Y":dbl, "PZT_Z":dbl})
              n153 = Not(x=w426) -> (.not. x?=w425:bool)
            }
            event "PZT_X-": Value Change {
              n154 = event-data() -> ()  [unwired: 1 in, 1 out]
              n155 = Wait (ms)(milliseconds to wait=w435) -> ()  [unwired: 1 out]
              n156 = local read "PZT_Step"() -> (w434:dbl)
              n157 = Unbundle By Name(w442) -> ("PZT_X"=w444:dbl)
              n158 = Add(x=w444, y=w434) -> (x+y=w439:dbl)
              n159 = In Range and Coerce(upper limit=5000.0, x=w439, lower limit=-5000.0) -> (coerced(x)=w437:dbl, In Range?=w440:bool)
              n160 = Bundle By Name(cluster=w442, "PZT_X"=w437) -> (w443:cluster{"PZT_X":dbl, "PZT_Y":dbl, "PZT_Z":dbl})
              n161 = Not(x=w440) -> (.not. x?=w438:bool)
            }
            event "PZT_Y+": Value Change {
              n162 = event-data() -> ()  [unwired: 1 in, 1 out]
              n163 = Wait (ms)(milliseconds to wait=w446) -> ()  [unwired: 1 out]
              n164 = local read "PZT_Step"() -> (w445:dbl)
              n165 = Unbundle By Name(w453) -> ("PZT_Y"=w455:dbl)
              n166 = Add(x=w455, y=w445) -> (x+y=w450:dbl)
              n167 = In Range and Coerce(upper limit=5000.0, x=w450, lower limit=ext -5000.0) -> (coerced(x)=w449:ext, In Range?=w451:bool)
              n168 = Bundle By Name(cluster=w453, "PZT_Y"=w449) -> (w454:cluster{"PZT_X":dbl, "PZT_Y":dbl, "PZT_Z":dbl})
              n169 = Not(x=w451) -> (.not. x?=w448:bool)
            }
            event "PZT_Y-": Value Change {
              n170 = event-data() -> ()  [unwired: 1 in, 1 out]
              n171 = Wait (ms)(milliseconds to wait=w457) -> ()  [unwired: 1 out]
              n172 = local read "PZT_Step"() -> (w456:dbl)
              n173 = Unbundle By Name(w464) -> ("PZT_Y"=w466:dbl)
              n174 = Subtract(x=w466, y=w456) -> (x-y=w459:dbl)
              n175 = In Range and Coerce(upper limit=5000.0, x=w459, lower limit=-5000.0) -> (coerced(x)=w458:dbl, In Range?=w462:bool)
              n176 = Bundle By Name(cluster=w464, "PZT_Y"=w458) -> (w465:cluster{"PZT_X":dbl, "PZT_Y":dbl, "PZT_Z":dbl})
              n177 = Not(x=w462) -> (.not. x?=w461:bool)
            }
            event "PZT_Z+": Value Change {
              n178 = event-data() -> ()  [unwired: 1 in, 1 out]
              n179 = Wait (ms)(milliseconds to wait=w468) -> ()  [unwired: 1 out]
              n180 = local read "PZT_Step"() -> (w467:dbl)
              n181 = Unbundle By Name(w475) -> ("PZT_Z"=w477:dbl)
              n182 = Subtract(x=w477, y=w467) -> (x-y=w472:dbl)
              n183 = In Range and Coerce(upper limit=3000.0, x=w472, lower limit=-3000.0) -> (coerced(x)=w470:dbl, In Range?=w473:bool)
              n184 = Bundle By Name(cluster=w475, "PZT_Z"=w470) -> (w476:cluster{"PZT_X":dbl, "PZT_Y":dbl, "PZT_Z":dbl})
              n185 = Not(x=w473) -> (.not. x?=w469:bool)
            }
            event "PZT_Z-": Value Change {
              n186 = event-data() -> ()  [unwired: 1 in, 1 out]
              n187 = Wait (ms)(milliseconds to wait=w479) -> ()  [unwired: 1 out]
              n188 = local read "PZT_Step"() -> (w478:dbl)
              n189 = Unbundle By Name(w486) -> ("PZT_Z"=w488:dbl)
              n190 = Add(x=w488, y=w478) -> (x+y=w483:dbl)
              n191 = In Range and Coerce(upper limit=3000.0, x=w483, lower limit=-3000.0) -> (coerced(x)=w481:dbl, In Range?=w484:bool)
              n192 = Bundle By Name(cluster=w486, "PZT_Z"=w481) -> (w487:cluster{"PZT_X":dbl, "PZT_Y":dbl, "PZT_Z":dbl})
              n193 = Not(x=w484) -> (.not. x?=w480:bool)
            }
            event "PZT_Center": Value Change {
              w489 = 0.0 ("PZT_X")
              n194 = event-data() -> ()  [unwired: 1 in, 1 out]
              n195 = Wait (ms)(milliseconds to wait=w490) -> ()  [unwired: 1 out]
              n196 = Bundle By Name(cluster=w492, "PZT_X"=w489, "PZT_Y"=w489, "PZT_Z"=w489) -> (w491:cluster{"PZT_X":dbl, "PZT_Y":dbl, "PZT_Z":dbl})
            }
            event "PZT_Move": Value Change {
              n197 = event-data() -> ()  [unwired: 1 in, 1 out]
              n198 = Wait (ms)(milliseconds to wait=w493) -> ()  [unwired: 1 out]
              n199 = Bundle By Name(cluster=w498, "PZT_X"="PZTX_move", "PZT_Y"="PZTY_move", "PZT_Z"="PZTZ_move") -> (w497:cluster{"PZT_X":dbl, "PZT_Y":dbl, "PZT_Z":dbl})
            }
            event Key Down {
              n200 = event-data() -> ("VKey"=w503:T1)  [unwired: 1 in]
              n201 = Wait (ms)(milliseconds to wait=w499) -> ()  [unwired: 1 out]
              n202 = case shown="\"Left\"" w503 {
                tunnel: w502 -> [w512 w522 w532 w542 w552 w562 w566 w568]
                tunnel: [w511 w521 w531 w541 w551 w561 w566 w568] -> w501
                tunnel: [w506 w517 w527 w537 w547 w557 FALSE FALSE] -> w500
                frame "Up" {
                  n203 = local read "PZT_Step"() -> (w504:dbl)
                  n204 = Unbundle By Name(w512) -> ("PZT_Y"=w513:dbl)
                  n205 = Add(x=w513, y=w504) -> (x+y=w508:dbl)
                  n206 = In Range and Coerce(upper limit=5000.0, x=w508, lower limit=-5000.0) -> (coerced(x)=w505:dbl, In Range?=w509:bool)
                  n207 = Bundle By Name(cluster=w512, "PZT_Y"=w505) -> (w511:cluster{"PZT_X":dbl, "PZT_Y":dbl, "PZT_Z":dbl})
                  n208 = Not(x=w509) -> (.not. x?=w506:bool)
                }
                frame "Down" {
                  n209 = local read "PZT_Step"() -> (w514:dbl)
                  n210 = Unbundle By Name(w522) -> ("PZT_Y"=w523:dbl)
                  n211 = Subtract(x=w523, y=w514) -> (x-y=w516:dbl)
                  n212 = In Range and Coerce(upper limit=5000.0, x=w516, lower limit=-5000.0) -> (coerced(x)=w515:dbl, In Range?=w519:bool)
                  n213 = Bundle By Name(cluster=w522, "PZT_Y"=w515) -> (w521:cluster{"PZT_X":dbl, "PZT_Y":dbl, "PZT_Z":dbl})
                  n214 = Not(x=w519) -> (.not. x?=w517:bool)
                }
                frame "Left" {
                  n215 = local read "PZT_Step"() -> (w524:dbl)
                  n216 = Unbundle By Name(w532) -> ("PZT_X"=w533:dbl)
                  n217 = Add(x=w533, y=w524) -> (x+y=w526:dbl)
                  n218 = In Range and Coerce(upper limit=5000.0, x=w526, lower limit=ext -5000.0) -> (coerced(x)=w525:ext, In Range?=w529:bool)
                  n219 = Bundle By Name(cluster=w532, "PZT_X"=w525) -> (w531:cluster{"PZT_X":dbl, "PZT_Y":dbl, "PZT_Z":dbl})
                  n220 = Not(x=w529) -> (.not. x?=w527:bool)
                }
                frame "Right" {
                  n221 = local read "PZT_Step"() -> (w534:dbl)
                  n222 = Unbundle By Name(w542) -> ("PZT_X"=w543:dbl)
                  n223 = Subtract(x=w543, y=w534) -> (x-y=w536:dbl)
                  n224 = In Range and Coerce(upper limit=5000.0, x=w536, lower limit=-5000.0) -> (coerced(x)=w535:dbl, In Range?=w539:bool)
                  n225 = Bundle By Name(cluster=w542, "PZT_X"=w535) -> (w541:cluster{"PZT_X":dbl, "PZT_Y":dbl, "PZT_Z":dbl})
                  n226 = Not(x=w539) -> (.not. x?=w537:bool)
                }
                frame "PageUp" {
                  n227 = local read "PZT_Step"() -> (w544:dbl)
                  n228 = Unbundle By Name(w552) -> ("PZT_Z"=w553:dbl)
                  n229 = Subtract(x=w553, y=w544) -> (x-y=w546:dbl)
                  n230 = In Range and Coerce(upper limit=3000.0, x=w546, lower limit=-3000.0) -> (coerced(x)=w545:dbl, In Range?=w549:bool)
                  n231 = Bundle By Name(cluster=w552, "PZT_Z"=w545) -> (w551:cluster{"PZT_X":dbl, "PZT_Y":dbl, "PZT_Z":dbl})
                  n232 = Not(x=w549) -> (.not. x?=w547:bool)
                }
                frame "PageDown" {
                  n233 = local read "PZT_Step"() -> (w554:dbl)
                  n234 = Unbundle By Name(w562) -> ("PZT_Z"=w563:dbl)
                  n235 = Add(x=w563, y=w554) -> (x+y=w556:dbl)
                  n236 = In Range and Coerce(upper limit=3000.0, x=w556, lower limit=-3000.0) -> (coerced(x)=w555:dbl, In Range?=w559:bool)
                  n237 = Bundle By Name(cluster=w562, "PZT_Z"=w555) -> (w561:cluster{"PZT_X":dbl, "PZT_Y":dbl, "PZT_Z":dbl})
                  n238 = Not(x=w559) -> (.not. x?=w557:bool)
                }
                frame "Ctrl" {
                  n239 = local read "PZT_manual"() -> (w565:bool)
                  n240 = local write "PZT_oscillation"(w565) -> ()
                }
                frame Default {
                }
              }
            }
            event Panel Close {
              n241 = event-data() -> ()  [unwired: 1 in, 1 out]
              n242 = Unbundle By Name(w569) -> ("PZT_X"=w573:dbl, "PZT_Y"=w572:dbl, "PZT_Z"=w571:dbl)
              n243 = Build Array(w573, w572, w571) -> (w570:dbl[])
              n244 = call "Convert to Dynamic Data2"("Array"=w570) -> ("Dynamic Data Type"=w574:dynamicdata)  [unwired: 3 in]
              n245 = call "Write To Measurement File2"("Signals"=w574) -> ()  [unwired: 16 in, 3 out]
            }
            event Application Instance Close {
              n246 = event-data() -> ()  [unwired: 1 in, 1 out]
              n247 = Unbundle By Name(w575) -> ("PZT_X"=w579:dbl, "PZT_Y"=w578:dbl, "PZT_Z"=w577:dbl)
              n248 = Build Array(w579, w578, w577) -> (w576:dbl[])
              n249 = call "Convert to Dynamic Data3"("Array"=w576) -> ("Dynamic Data Type"=w580:dynamicdata)  [unwired: 3 in]
              n250 = call "Write To Measurement File3"("Signals"=w580) -> ()  [unwired: 16 in, 3 out]
            }
            event Key Repeat {
              n251 = event-data() -> ("VKey"=w585:T1)  [unwired: 1 in]
              n252 = Wait (ms)(milliseconds to wait=w581) -> ()  [unwired: 1 out]
              n253 = case shown="\"Up\"" w585 {
                tunnel: w584 -> [w594 w604 w614 w624 w634 w644 w647]
                tunnel: [w593 w603 w613 w623 w633 w643 w647] -> w583
                tunnel: [w587 w597 w607 w617 w627 w637 FALSE] -> w582
                frame "Up" {
                  n254 = local read "PZT_Step"() -> (w586:dbl)
                  n255 = Unbundle By Name(w594) -> ("PZT_Y"=w595:dbl)
                  n256 = Add(x=w595, y=w586) -> (x+y=w592:dbl)
                  n257 = In Range and Coerce(upper limit=5000.0, x=w592, lower limit=-5000.0) -> (coerced(x)=w591:dbl, In Range?=w588:bool)
                  n258 = Bundle By Name(cluster=w594, "PZT_Y"=w591) -> (w593:cluster{"PZT_X":dbl, "PZT_Y":dbl, "PZT_Z":dbl})
                  n259 = Not(x=w588) -> (.not. x?=w587:bool)
                }
                frame "Down" {
                  n260 = local read "PZT_Step"() -> (w596:dbl)
                  n261 = Unbundle By Name(w604) -> ("PZT_Y"=w605:dbl)
                  n262 = Subtract(x=w605, y=w596) -> (x-y=w602:dbl)
                  n263 = In Range and Coerce(upper limit=5000.0, x=w602, lower limit=-5000.0) -> (coerced(x)=w599:dbl, In Range?=w598:bool)
                  n264 = Bundle By Name(cluster=w604, "PZT_Y"=w599) -> (w603:cluster{"PZT_X":dbl, "PZT_Y":dbl, "PZT_Z":dbl})
                  n265 = Not(x=w598) -> (.not. x?=w597:bool)
                }
                frame "Left" {
                  n266 = local read "PZT_Step"() -> (w606:dbl)
                  n267 = Unbundle By Name(w614) -> ("PZT_X"=w615:dbl)
                  n268 = Add(x=w615, y=w606) -> (x+y=w612:dbl)
                  n269 = In Range and Coerce(upper limit=5000.0, x=w612, lower limit=-5000.0) -> (coerced(x)=w609:dbl, In Range?=w608:bool)
                  n270 = Bundle By Name(cluster=w614, "PZT_X"=w609) -> (w613:cluster{"PZT_X":dbl, "PZT_Y":dbl, "PZT_Z":dbl})
                  n271 = Not(x=w608) -> (.not. x?=w607:bool)
                }
                frame "Right" {
                  n272 = local read "PZT_Step"() -> (w616:dbl)
                  n273 = Unbundle By Name(w624) -> ("PZT_X"=w625:dbl)
                  n274 = Subtract(x=w625, y=w616) -> (x-y=w622:dbl)
                  n275 = In Range and Coerce(upper limit=5000.0, x=w622, lower limit=-5000.0) -> (coerced(x)=w619:dbl, In Range?=w618:bool)
                  n276 = Bundle By Name(cluster=w624, "PZT_X"=w619) -> (w623:cluster{"PZT_X":dbl, "PZT_Y":dbl, "PZT_Z":dbl})
                  n277 = Not(x=w618) -> (.not. x?=w617:bool)
                }
                frame "PageUp" {
                  n278 = local read "PZT_Step"() -> (w626:dbl)
                  n279 = Unbundle By Name(w634) -> ("PZT_Z"=w635:dbl)
                  n280 = Subtract(x=w635, y=w626) -> (x-y=w632:dbl)
                  n281 = In Range and Coerce(upper limit=3000.0, x=w632, lower limit=-3000.0) -> (coerced(x)=w629:dbl, In Range?=w628:bool)
                  n282 = Bundle By Name(cluster=w634, "PZT_Z"=w629) -> (w633:cluster{"PZT_X":dbl, "PZT_Y":dbl, "PZT_Z":dbl})
                  n283 = Not(x=w628) -> (.not. x?=w627:bool)
                }
                frame "PageDown" {
                  n284 = local read "PZT_Step"() -> (w636:dbl)
                  n285 = Unbundle By Name(w644) -> ("PZT_Z"=w645:dbl)
                  n286 = Add(x=w645, y=w636) -> (x+y=w642:dbl)
                  n287 = In Range and Coerce(upper limit=3000.0, x=w642, lower limit=-3000.0) -> (coerced(x)=w639:dbl, In Range?=w638:bool)
                  n288 = Bundle By Name(cluster=w644, "PZT_Z"=w639) -> (w643:cluster{"PZT_X":dbl, "PZT_Y":dbl, "PZT_Z":dbl})
                  n289 = Not(x=w638) -> (.not. x?=w637:bool)
                }
                frame Default {
                }
              }
            }
          }
          "PZT_Caution" <- w335
          n290 = Unbundle By Name(w331) -> ("PZT_X"=w328:dbl, "PZT_Y"=w315:dbl, "PZT_Z"=w330:dbl)
          "PZT_Y" <- w315
          n291 = Negate(x=w328) -> (-x=→"PZT_X":dbl)
          n292 = Negate(x=w330) -> (-x=→"PZT_Z":dbl)
          n293 = Add(x=w328, y=w322) -> (x+y=w326:dbl)
          n294 = Add(x=w322, y=w315) -> (x+y=w325:dbl)
          n295 = Add(x=w330, y=15000.0) -> (x+y=w324:dbl)
          n296 = global write "PZT_oscillation.vi" "PZT_oscillation"("PZT_oscillation") -> ()
          n297 = Divide(x=w326, y=w334) -> (x/y=w321:dbl)
          "PZTX_Vin" <- w321
          n298 = Divide(x=w325, y=w334) -> (x/y=w320:dbl)
          "PZTY_Vin" <- w320
          n299 = Divide(x=w324, y=3000.0) -> (x/y=w319:dbl)
          "PZTZ_Vin" <- w319
          n300 = case shown="True" "PZT_oscillation" {
            selector: "PZT_oscillation" -> [w352 w357]
            tunnel: [w338 w362] -> w317
            tunnel: w321 -> [w344 w356]
            tunnel: w320 -> [w343 w355]
            tunnel: w319 -> [w342 w354]
            frame False {
              n301 = Not(x=w352) -> (.not. x?=w353:bool)
              n302 = local write "PZT_manual"(w353) -> ()
              n303 = Build Array(w344, w343, w342) -> (w341:dbl[])
              n304 = call-poly <vilib>:"DAQmx Create Virtual Channel.vi"("maximum value"=6.0, "minimum value"=4.0, "physical channels"=tag "DAQ/ao0:2") -> ("task out"=w348:refnum<k21>, "error out"=w347:errorcluster)  [unwired: 11 in]
              n305 = call <vilib>:"DAQmx Start Task.vi"("task/channels in"=w348, "error in"=w347) -> ("task out"=w346:refnum<k21>, "error out"=w345:errorcluster)  [unwired: 12 in]
              n306 = call-poly <vilib>:"DAQmx Write.vi"("task/channels in"=w346, "data"=w341, "error in"=w345) -> ("task out"=w340:refnum<k21>, "error out"=w339:errorcluster)  [unwired: 10 in, 1 out]
              n307 = call <vilib>:"DAQmx Clear Task.vi"("task in"=w340, "error in"=w339) -> ("error out"=w338:errorcluster)  [unwired: 13 in]
            }
            frame True {
              n308 = Not(x=w357) -> (.not. x?=→"PZT_manual":bool)
              n309 = case shown="\"X-axis\", Default" "PZT_Axis" {
                tunnel: [w370 w384 w408] -> w362
                tunnel: "PZT_Waveform" -> [w365 w388 w406]
                tunnel: "PZT_Frequency" -> [w369 w389 w407]
                tunnel: "PZT_Amplitude" -> [w368 w385 w404]
                tunnel: w356 -> [w364 _ _]
                tunnel: w355 -> [_ w383 _]
                tunnel: w354 -> [_ _ w402]
                frame "X-axis", Default {
                  n310 = Divide(x=w368, y=5000.0) -> (x/y=w367:dbl)
                  n311 = call "PZT_SignalGenerator.vi"("Waveform Type"=w365, "Physical Channels"=tag "DAQ/ao0", "Offset"=w364, "Frequency"=w369, "Amplitude"=w367) -> ("error out"=w370:errorcluster)  [unwired: 2 in, 1 out]
                  n312 = while {
                    i -> [w375]
                    stop <- w374 stop-if-true
                    n313 = local read "PZT_oscillation"() -> (w373:bool)
                    n314 = global write "PZT_oscillation.vi" "PZT_oscillation"(w373) -> ()
                    n315 = event shown="[1] Key Down" {
                      selector: _ -> [_ _]
                      dyn-events: _ -> [_ _]
                      timeout: 10 -> [_ _]
                      event Timeout {
                        n316 = event-data() -> ()  [unwired: 1 in, 1 out]
                      }
                      event Key Down {
                        n317 = event-data() -> ("VKey"=w382:T1)  [unwired: 1 in]
                        n318 = local read "PZT_os_num"() -> (w378:i32)
                        n319 = Equal?(x=w382, y=eventvkey."Ctrl") -> (x = y?=w380:bool)
                        n320 = Greater Than 0?(x=w378) -> (x > 0?=w379:bool)
                        n321 = Not And(1:w379, 2:w380) -> (0:w377:bool)
                        n322 = local write "PZT_oscillation"(w377) -> ()
                      }
                    }
                    n323 = Not(x=w373) -> (.not. x?=w374:bool)
                    n324 = Wait (ms)(milliseconds to wait=u32 10) -> ()  [unwired: 1 out]
                    "PZT_os_num" <- w375
                  }
                }
                frame "Y-axis" {
                  n325 = Divide(x=w385, y=5000.0) -> (x/y=w386:dbl)
                  n326 = call "PZT_SignalGenerator.vi"("Waveform Type"=w388, "Physical Channels"=tag "DAQ/ao1", "Offset"=w383, "Frequency"=w389, "Amplitude"=w386) -> ("error out"=w384:errorcluster)  [unwired: 2 in, 1 out]
                  n327 = while {
                    i -> [w394]
                    stop <- w393 stop-if-true
                    n328 = local read "PZT_oscillation"() -> (w392:bool)
                    n329 = global write "PZT_oscillation.vi" "PZT_oscillation"(w392) -> ()
                    n330 = event shown="[1] Key Down" {
                      selector: _ -> [_ _]
                      dyn-events: _ -> [_ _]
                      timeout: 10 -> [_ _]
                      event Timeout {
                        n331 = event-data() -> ()  [unwired: 1 in, 1 out]
                      }
                      event Key Down {
                        n332 = event-data() -> ("VKey"=w401:T1)  [unwired: 1 in]
                        n333 = local read "PZT_os_num"() -> (w397:i32)
                        n334 = Equal?(x=w401, y=eventvkey."Ctrl") -> (x = y?=w399:bool)
                        n335 = Greater Than 0?(x=w397) -> (x > 0?=w398:bool)
                        n336 = Not And(1:w398, 2:w399) -> (0:w396:bool)
                        n337 = local write "PZT_oscillation"(w396) -> ()
                      }
                    }
                    n338 = local write "PZT_os_num"(w394) -> ()
                    n339 = Not(x=w392) -> (.not. x?=w393:bool)
                    n340 = Wait (ms)(milliseconds to wait=u32 100) -> ()  [unwired: 1 out]
                  }
                }
                frame "Z-axis" {
                  n341 = Divide(x=w404, y=3000.0) -> (x/y=w403:dbl)
                  n342 = call "PZT_SignalGenerator.vi"("Waveform Type"=w406, "Physical Channels"=tag "DAQ/ao2", "Offset"=w402, "Frequency"=w407, "Amplitude"=w403) -> ("error out"=w408:errorcluster)  [unwired: 2 in, 1 out]
                  n343 = while {
                    i -> [w411]
                    stop <- w413 stop-if-true
                    n344 = local read "PZT_oscillation"() -> (w412:bool)
                    n345 = global write "PZT_oscillation.vi" "PZT_oscillation"(w412) -> ()
                    n346 = event shown="[1] Key Down" {
                      selector: _ -> [_ _]
                      dyn-events: _ -> [_ _]
                      timeout: 10 -> [_ _]
                      event Timeout {
                        n347 = event-data() -> ()  [unwired: 1 in, 1 out]
                      }
                      event Key Down {
                        n348 = event-data() -> ("VKey"=w420:T1)  [unwired: 1 in]
                        n349 = local read "PZT_os_num"() -> (w416:i32)
                        n350 = Equal?(x=w420, y=eventvkey."Ctrl") -> (x = y?=w418:bool)
                        n351 = Greater Than 0?(x=w416) -> (x > 0?=w417:bool)
                        n352 = Not And(1:w417, 2:w418) -> (0:w415:bool)
                        n353 = local write "PZT_oscillation"(w415) -> ()
                      }
                    }
                    n354 = Not(x=w412) -> (.not. x?=w413:bool)
                    n355 = local write "PZT_os_num"(w411) -> ()
                    n356 = Wait (ms)(milliseconds to wait=u32 100) -> ()  [unwired: 1 out]
                  }
                }
              }
            }
          }
          n357 = Or(x="PZT_STOP", y=w317) -> (x .or. y?=w327:bool)
          "PZT_man_num" <- w337
        }
      }
    }
    n358 = Merge Errors(w299, w298) -> (w294:errorcluster)
    n359 = local write "PZT_manual"(FALSE) -> ()
    n360 = Unbundle By Name(w294) -> ("status"=w293:bool)
    "PZT_Error" <- w293
    n361 = Or(x="STOP", y=w293) -> (x .or. y?=w300:bool)
    n362 = Wait (ms)(milliseconds to wait=u32 100) -> ()  [unwired: 1 out]
    "PZT_ON" <- "PZT_START"
  }
  n363 = while {
    tunnel: w2 -> [w648]
    tunnel: [w653] -> w10
    stop <- w650 stop-if-true
    # "Fluorescence Laser"
    n364 = case shown="True" "OK Button 6" {
      tunnel: [errorcluster {"status"=FALSE, "code"=0, "source"=""} ("error out") w657] -> w652
      frame False {
      }
      frame True {
        n365 = while "Event Handle Loop" {
          tunnel: [w658] -> w657
          i -> [w674]
          stop <- w663 stop-if-true
          w672 = 0 items=["one channel for each line", "one channel for all lines"] ("line grouping")
          # "Fluorescence Laser"
          n366 = Build Array("Flu_Blue", "Flu_Green", "Flu_Red") -> (w659:bool[])
          n367 = Wait (ms)(milliseconds to wait=u32 100) -> ()  [unwired: 1 out]
          n368 = call-poly <vilib>:"DAQmx Create Virtual Channel.vi"("lines"=tag "DAQ/port0/line0:2", "line grouping"=w672) -> ("task out"=w670:refnum<k21>, "error out"=w669:errorcluster)  [unwired: 12 in]
          n369 = call <vilib>:"DAQmx Start Task.vi"("task/channels in"=w670, "error in"=w669) -> ("task out"=w668:refnum<k21>, "error out"=w667:errorcluster)  [unwired: 12 in]
          n370 = call-poly <vilib>:"DAQmx Write.vi"("task/channels in"=w668, "data"=w659, "error in"=w667) -> ("task out"=w666:refnum<k21>, "error out"=w665:errorcluster)  [unwired: 10 in, 1 out]
          n371 = call <vilib>:"DAQmx Clear Task.vi"("task in"=w666, "error in"=w665) -> ("error out"=w658:errorcluster)  [unwired: 13 in]
          n372 = Or(x=w658, y="stop 6") -> (x .or. y?=w663:bool)
          "Numeric 9" <- w674
        }
      }
    }
    n373 = local read "STOP"() -> (w651:bool)
    n374 = Unbundle By Name(w652) -> ("status"=w649:bool)
    "PZT_Error 3" <- w649
    n375 = Merge Errors(w652, w648) -> (w653:errorcluster)
    n376 = Wait (ms)(milliseconds to wait=u32 100) -> ()  [unwired: 1 out]
    n377 = Or(x=w651, y=w649) -> (x .or. y?=w650:bool)
    "OK Button 10" <- "OK Button 6"
  }
  n378 = while {
    tunnel: w2 -> [w675]
    tunnel: [w680] -> w11
    stop <- w679 stop-if-true
    # "Stage-X"
    n379 = case shown="True" "StageX_Start" {
      tunnel: [errorcluster {"status"=FALSE, "code"=0, "source"=""} ("error out") w686] -> w676
      frame False {
      }
      frame True {
        n380 = call <userlib>:"Connect Newport Instrument1.vi"("Controller address"=1, "Selected device"="ASRL3  (COM3 - USB Serial Port)" ("String")) -> ("Connected"=w689:bool, "Device Connection Cluster"=w690:T3)  [unwired: 5 in, 3 out]
        n381 = case shown="True" w689 {
          tunnel: w690 -> [w692 w695]
          tunnel: [w692 w697] -> w688
          tunnel: [errorcluster {"status"=FALSE, "code"=0, "source"=""} ("error IO") w696] -> w686
          frame False {
          }
          frame True {
            # "x = [0-5]\nv = [0.1-2]"
            n382 = call <userlib>:"CONEX-CC Set Negative Software Limit v2.vi"("Negative limit (left)"=0.0, "Connection Cluster in"=w695) -> ("Connection Cluster out"=w701:T3)  [unwired: 9 in]
            n383 = call <userlib>:"CONEX-CC Set Positive Software Limit v2.vi"("Positive limit (right)"=5.0, "Connection Cluster in"=w701) -> ("Connection Cluster out"=w700:T3)  [unwired: 9 in]
            n384 = call <userlib>:"CONEX-CC Set Velocity v2.vi"("Velocity"=1.0, "Connection Cluster in"=w700) -> ("Connection Cluster out"=w694:T3)  [unwired: 9 in]
            n385 = while {
              shift-right: [w706] -> w697
              shift-left: w694 -> [w705]
              tunnel: [w719] -> w696
              i -> [w721]
              stop <- w716 stop-if-true
              w713 = 2000.0 ("upper limit")
              n386 = Negate(x=w713) -> (-x=w714:dbl)
              n387 = call <userlib>:"CONEX-CC Get Current Position v2.vi"("Connection Cluster in"=w705) -> ("Current position"=w707:dbl, "Connection Cluster out"=w703:T3)  [unwired: 8 in, 1 out]
              n388 = Subtract(x=w707, y=2.5) -> (x-y=w709:dbl)
              n389 = Multiply(x=w709, y=1000.0) -> (x*y=w712:dbl)
              "StageX_Position" <- w712
              n390 = In Range and Coerce(upper limit=w713, x=w712, lower limit=w714) -> (In Range?=w711:bool)  [unwired: 1 out]
              n391 = Not(x=w711) -> (.not. x?=→"StageX_Limit":bool)
              n392 = call <userlib>:"CONEX-CC Get Velocity v2.vi"("Connection Cluster in"=w703) -> ("Connection Cluster out"=w702:T3)  [unwired: 8 in, 2 out]
              n393 = case shown="False" "Stage_Step_Select" {
                frame False {
                  n394 = local write "StageX_Step"("StageX_Step1") -> ()
                }
                frame True {
                  "StageX_Step" <- "StageX_Step2"
                }
              }
              n395 = event shown="[5] \"StageX_Home\": Value Change" {
                selector: _ -> [_ _ _ _ _ _ _]
                dyn-events: _ -> [_ _ _ _ _ _ _]
                timeout: 10 -> [_ _ _ _ _ _ _]
                tunnel: w702 -> [w726 w727 w737 w744 w773 w799 w821]
                tunnel: [w726 w731 w734 w743 w772 w792 w821] -> w706
                event Timeout {
                  n396 = event-data() -> ()  [unwired: 1 in, 1 out]
                }
                event "StageX+": Value Change {
                  n397 = event-data() -> ()  [unwired: 1 in, 1 out]
                  n398 = local read "StageX_Step"() -> (w728:dbl)
                  n399 = Divide(x=w728, y=1000.0) -> (x/y=w730:dbl)
                  n400 = call <userlib>:"CONEX-CC Relative Move v2.vi"("Relative displacement"=w730, "Connection Cluster in"=w727) -> ("Connection Cluster out"=w731:T3)  [unwired: 9 in]
                }
                event "StageX-": Value Change {
                  n401 = event-data() -> ()  [unwired: 1 in, 1 out]
                  n402 = local read "StageX_Step"() -> (w736:dbl)
                  n403 = Negate(x=w736) -> (-x=w735:dbl)
                  n404 = Divide(x=w735, y=1000.0) -> (x/y=w733:dbl)
                  n405 = call <userlib>:"CONEX-CC Relative Move v2.vi"("Relative displacement"=w733, "Connection Cluster in"=w737) -> ("Connection Cluster out"=w734:T3)  [unwired: 9 in]
                }
                event Key Down {
                  n406 = event-data() -> ("Char"=w739:i16, "ScanCode"=w738:i16)  [unwired: 1 in]
                  n407 = local read "StageX_Step"() -> (w741:dbl)
                  n408 = Divide(x=w741, y=1000.0) -> (x/y=w740:dbl)
                  n409 = case shown="53" w739 {
                    tunnel: w744 -> [w745 w749 w758 w764]
                    tunnel: [w745 w748 w757 w764] -> w743
                    tunnel: w740 -> [_ w747 w756 _]
                    tunnel: w738 -> [_ w746 w755 w763]
                    frame 0, Default {
                    }
                    frame 52 {
                      n410 = case shown="75" w746 {
                        tunnel: w749 -> [w750 w754]
                        tunnel: [w750 w753] -> w748
                        tunnel: w747 -> [_ w752]
                        frame 0, Default {
                        }
                        frame 75 {
                          n411 = Negate(x=w752) -> (-x=w751:dbl)
                          n412 = call <userlib>:"CONEX-CC Relative Move v2.vi"("Relative displacement"=w751, "Connection Cluster in"=w754) -> ("Connection Cluster out"=w753:T3)  [unwired: 9 in]
                        }
                      }
                    }
                    frame 54 {
                      n413 = case shown="77" w755 {
                        tunnel: w758 -> [w759 w762]
                        tunnel: [w759 w761] -> w757
                        tunnel: w756 -> [_ w760]
                        frame 0, Default {
                        }
                        frame 77 {
                          n414 = call <userlib>:"CONEX-CC Relative Move v2.vi"("Relative displacement"=w760, "Connection Cluster in"=w762) -> ("Connection Cluster out"=w761:T3)  [unwired: 9 in]
                        }
                      }
                    }
                    frame 53 {
                      n415 = case shown="76" w763 {
                        frame 0, Default {
                        }
                        frame 76 {
                          n416 = local read "Stage_Step_Select"() -> (w765:bool)
                          n417 = Not(x=w765) -> (.not. x?=w766:bool)
                          n418 = local write "Stage_Step_Select"(w766) -> ()
                        }
                      }
                    }
                  }
                }
                event Key Repeat {
                  n419 = event-data() -> ("Char"=w771:i16, "ScanCode"=w767:i16)  [unwired: 1 in]
                  n420 = local read "StageX_Step"() -> (w769:dbl)
                  n421 = Divide(x=w769, y=1000.0) -> (x/y=w768:dbl)
                  n422 = case shown="52" w771 {
                    tunnel: w773 -> [w774 w778 w787]
                    tunnel: [w774 w777 w786] -> w772
                    tunnel: w768 -> [_ w776 w785]
                    tunnel: w767 -> [_ w775 w784]
                    frame 0, Default {
                    }
                    frame 52 {
                      n423 = case shown="75" w775 {
                        tunnel: w778 -> [w779 w783]
                        tunnel: [w779 w782] -> w777
                        tunnel: w776 -> [_ w781]
                        frame 0, Default {
                        }
                        frame 75 {
                          n424 = Negate(x=w781) -> (-x=w780:dbl)
                          n425 = call <userlib>:"CONEX-CC Relative Move v2.vi"("Relative displacement"=w780, "Connection Cluster in"=w783) -> ("Connection Cluster out"=w782:T3)  [unwired: 9 in]
                        }
                      }
                    }
                    frame 54 {
                      n426 = case shown="77" w784 {
                        tunnel: w787 -> [w788 w791]
                        tunnel: [w788 w790] -> w786
                        tunnel: w785 -> [_ w789]
                        frame 0, Default {
                        }
                        frame 77 {
                          n427 = call <userlib>:"CONEX-CC Relative Move v2.vi"("Relative displacement"=w789, "Connection Cluster in"=w791) -> ("Connection Cluster out"=w790:T3)  [unwired: 9 in]
                        }
                      }
                    }
                  }
                }
                event "StageX_Home": Value Change {
                  n428 = event-data() -> ()  [unwired: 1 in, 1 out]
                  n429 = call <userlib>:"CONEX-CC Set Velocity v2.vi"("Velocity"=0.1, "Connection Cluster in"=w799) -> ("Connection Cluster out"=w798:T3)  [unwired: 9 in]
                  n430 = call <userlib>:"CONEX-CC Absolute Move v2.vi"("Target position"=2.5, "Connection Cluster in"=w798) -> ("Connection Cluster out"=w795:T3)  [unwired: 5 in, 2 out]
                  n431 = while {
                    shift-right: [w800] -> w793
                    shift-left: w795 -> [w804]
                    stop <- w802 stop-if-true
                    n432 = flat-sequence {
                      tunnel: w804 -> [w812]
                      tunnel: [w811] -> w803
                      tunnel: [w810] -> w801
                      tunnel: w803 -> [w816]
                      tunnel: [w816] -> w802
                      tunnel: w801 -> [w815]
                      tunnel: [w815] -> w800
                      frame #0 {
                        n433 = call <userlib>:"CONEX-CC Get Current Position v2.vi"("Connection Cluster in"=w812) -> ("Current position"=w809:dbl, "Connection Cluster out"=w810:T3)  [unwired: 8 in, 1 out]
                        n434 = Subtract(x=w809, y=2.5) -> (x-y=w808:dbl)
                        n435 = Multiply(x=1000.0, y=w808) -> (x*y=w806:dbl)
                        n436 = local write "StageX_Position"(w806) -> ()
                        n437 = In Range and Coerce(upper limit=2.501 ("x"), x=w809, lower limit=2.499 ("x")) -> (In Range?=w811:bool)  [unwired: 1 out]
                      }
                      frame #1 {
                        n438 = Wait (ms)(milliseconds to wait=u32 100) -> ()  [unwired: 1 out]
                      }
                    }
                  }
                  n439 = call <userlib>:"CONEX-CC Set Velocity v2.vi"("Velocity"=1.0, "Connection Cluster in"=w793) -> ("Connection Cluster out"=w792:T3)  [unwired: 9 in]
                }
                event "Stage_Step_Select": Value Change {
                  n440 = event-data() -> ()  [unwired: 1 in, 1 out]
                  n441 = local read "Stage_Step_Select"() -> (w819:bool)
                  n442 = local read "StageX_Step1"() -> (w818:dbl)
                  n443 = local read "StageX_Step2"() -> (w820:dbl)
                  n444 = Select(t=w820, s=w819, f=w818) -> (s? t:f=w822:dbl)
                  n445 = local write "StageX_Step"(w822) -> ()
                }
              }
              n446 = Unbundle By Name(w706) -> ("error"=w719:errorcluster)
              n447 = Wait (ms)(milliseconds to wait=u32 100) -> ()  [unwired: 1 out]
              n448 = Unbundle By Name(w719) -> ("status"=w720:bool)
              n449 = Or(x=w720, y="StageX_Stop") -> (x .or. y?=w716:bool)
              n450 = Not(x=w716) -> (.not. x?=→"StageX_Connection":bool)
              "Numeric" <- w721
            }
          }
        }
        n451 = Unbundle By Name(w688) -> ("VISA resource name"=w687:refnum<visa-resource-name>)
        n452 = call <userlib>:"_Close Communications.vi"("Instrument Channel"=w687) -> ()  [unwired: 14 in, 1 out]
      }
    }
    n453 = local read "STOP"() -> (w678:bool)
    n454 = Unbundle By Name(w676) -> ("status"=w677:bool)
    "PZT_Error 4" <- w677
    n455 = Or(x=w678, y=w677) -> (x .or. y?=w679:bool)
    n456 = Merge Errors(w676, w675) -> (w680:errorcluster)
    n457 = Wait (ms)(milliseconds to wait=u32 100) -> ()  [unwired: 1 out]
  }
  n458 = while {
    tunnel: w2 -> [w824]
    tunnel: [w824] -> w5
    stop <- w825 stop-if-true
    # "Detection Laser"
    n459 = case shown="True" "OK Button 4" {
      frame False {
      }
      frame True {
        n460 = while "Event Handle Loop" {
          i -> [w829]
          stop <- "stop 4" stop-if-true
          # "Detection Laser"
          n461 = Wait (ms)(milliseconds to wait=u32 100) -> ()  [unwired: 1 out]
          n462 = event shown="[1] Key Down" {
            selector: _ -> [_ _]
            dyn-events: _ -> [_ _]
            timeout: 100 -> [_ _]
            event Timeout {
              n463 = event-data() -> ()  [unwired: 1 in, 1 out]
            }
            event Key Down {
              n464 = event-data() -> ()  [unwired: 1 in, 1 out]
            }
          }
          "Numeric 7" <- w829
        }
      }
    }
    n465 = local read "STOP"() -> (w825:bool)
    n466 = Wait (ms)(milliseconds to wait=u32 100) -> ()  [unwired: 1 out]
    "OK Button 8" <- "OK Button 4"
  }
  n467 = Merge Errors(w4, w1) -> (w3:errorcluster)
  n468 = Merge Errors(w11, w9, w3) -> (w7:errorcluster)
  n469 = Merge Errors(w29, w28, w10, w5) -> (w8:errorcluster)
  n470 = Merge Errors(w8, w7) -> (w6:errorcluster)
  n471 = call <vilib>:"Simple Error Handler.vi"("error in (no error)"=w6) -> ()  [unwired: 4 in, 5 out]
  n472 = Unbundle By Name(w15) -> ("PZT_X"=w18:dbl, "PZT_Y"=w17:dbl, "PZT_Z"=w16:dbl)
  n473 = Build Array(w18, w17, w16) -> (w14:dbl[])
  n474 = call "Convert to Dynamic Data"("Array"=w14) -> ("Dynamic Data Type"=w27:dynamicdata)  [unwired: 3 in]
  n475 = call "Write To Measurement File"("Signals"=w27) -> ()  [unwired: 16 in, 3 out]
